vi "set labels.vi"(0 "axis labels":string) -> (1 "axe x label":string, 2 "axe y label":string)   [LabVIEW 2013]
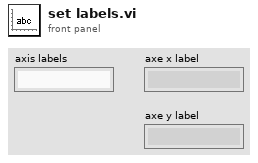
[diagram p1: front panel]
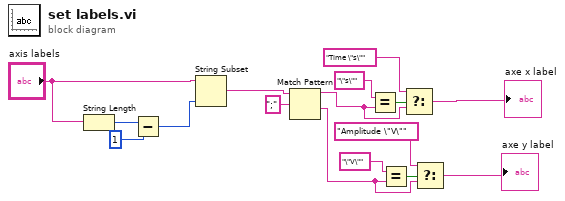
[diagram p0: block diagram]
diagram:
  n1 = String Length(string="axis labels") -> (length=w4:i32)
  n2 = Subtract(x=w4, y=1) -> (x-y=w2:i32)
  n3 = String Subset(string="axis labels", length (rest)=w2) -> (substring=w1:string)  [unwired: 1 in]
  n4 = Match Pattern(string=w1, regular expression=";") -> (before substring=w9:string, after substring=w16:string)  [unwired: 1 in, 2 out]
  n5 = Equal?(x="\"s\"" ("y"), y=w9) -> (x = y?=w7:bool)
  n6 = Equal?(x="\"V\"" ("y"), y=w16) -> (x = y?=w12:bool)
  n7 = Select(t="Time \"s\"", s=w7, f=w9) -> (s? t:f=→"axe x label":string)
  n8 = Select(t="Amplitude \"V\"", s=w12, f=w16) -> (s? t:f=→"axe y label":string)
